vi "Read INI Cluster.vi"(8 "error in (no error)":errorcluster, 10 "INI Fomatted Cluster Type":variant, 11 "refnum":T1) -> (0 "error out":errorcluster, 1 "all found?":bool, 2 "INI Fomatted Cluster":variant, 3 "dup refnum":T1, 4 "any found?":bool)   [LabVIEW 2020]
doc: "Reads a cluster of section formatted clusters from configuration data identified by refnum, and returns them as a cluster of clusters of items. Section cluster names are used as section names and key-value pairs correspond to the named cluster elements and thier values within the section formatted clusters. Only the section clusters and items within the \"INI Formatted Cluster Type\" input cluster are read from the configuration data and returned in the output cluster of clusters of items. The \"found?\" output will be TRUE only if all elements (recursively) are found.\n\nFor example an Cluster containins subClusters MyCluster1 and MyCluster2, where MyCluster1 contains two elements MyNumeric and MyBoolean, and MyCluster2 contains two elements MyEnum and MyString. This would correspond to an INI write of the following data:\n\n[MyCluster1]\nMyNumeric=1.024\nMyBoolean=TRUE\n[MyCluster2]\nMyEnum=init\nMyString=\"Hello World\"\n\nNote: Special characters in section and key names will be escape-coded. These include the following: \\00-\\1F (non-printable chars); \"[\", \"]\", and \"=\" (INI syntax elements); \\FE (\"þ\") and \\FF (\"ÿ\") (legacy bracket encoding); Additionally, the escape character, \"\\\", will be escaped as \"\\\\\".\n\nNote: This VI checks whether every element of the cluster has a name so it can be identified."
uses:
  <vilib>/Utility/config.llb/Config Data RefNum.ctl
  <vilib>/Utility/config.llb/NI_LVConfig.lvlib
panel:
  # "Read INI Cluster.vi\n\nReads a cluster (variant) of INI section clusters from INI file.\n\nPlease visit http://www.OpenG.org to learn about the\nOpen Source LabVIEW software movement.\n\nNOTICE -- YOU MUST LEAVE THIS NOTICE IN PLACE.  PER THE TERMS OF THE LICENSE BELOW, YOU MAY SUBLICENSE THIS SOFTWARE \nIN ANY WAY THAT DOES NOT CONFLICT WITH THIS LICENSE.\n\n### BSD License (http://www.opensource.org/licenses/bsd-license.php) Begin ###\n \nCopyright (c) 2002-2006, Jim Kring <jim@jimkring.com>\n\nAll rights reserved.\n\nRedistribution and use in source and binary forms, with or without modification, are permitted provided that the following conditions are met:\n\n    * Redistributions of source code must retain the above copyright notice, this list of conditions and the following disclaimer.\n    * Redistributions in binary form must reproduce the above copyright notice, this list of conditions and the following disclaimer in the \n       documentation and/or other materials provided with the distribution.\n    * Neither the name of SciWare, James Kring, Inc., nor the names of its contributors may be used to endorse or promote products derived \n       from this software without specific prior written permission.\n\nTHIS SOFTWARE IS PROVIDED BY THE COPYRIGHT HOLDERS AND CONTRIBUTORS \"AS IS\" AND ANY EXPRESS OR IMPLIED WARRANTIES, \nINCLUDING, BUT NOT LIMITED TO, THE IMPLIED WARRANTIES OF MERCHANTABILITY AND FITNESS FOR A PARTICULAR PURPOSE ARE \nDISCLAIMED. IN NO EVENT SHALL THE COPYRIGHT OWNER OR CONTRIBUTORS BE LIABLE FOR ANY DIRECT, INDIRECT, INCIDENTAL,\n SPECIAL, EXEMPLARY, OR CONSEQUENTIAL DAMAGES (INCLUDING, BUT NOT LIMITED TO, PROCUREMENT OF SUBSTITUTE GOODS OR \nSERVICES; LOSS OF USE, DATA, OR PROFITS; OR BUSINESS INTERRUPTION) HOWEVER CAUSED AND ON ANY THEORY OF LIABILITY, \nWHETHER IN CONTRACT, STRICT LIABILITY, OR TORT (INCLUDING NEGLIGENCE OR OTHERWISE) ARISING IN ANY WAY OUT OF THE USE \nOF THIS SOFTWARE, EVEN IF ADVISED OF THE POSSIBILITY OF SUCH DAMAGE.\n\n### BSD License End ###"
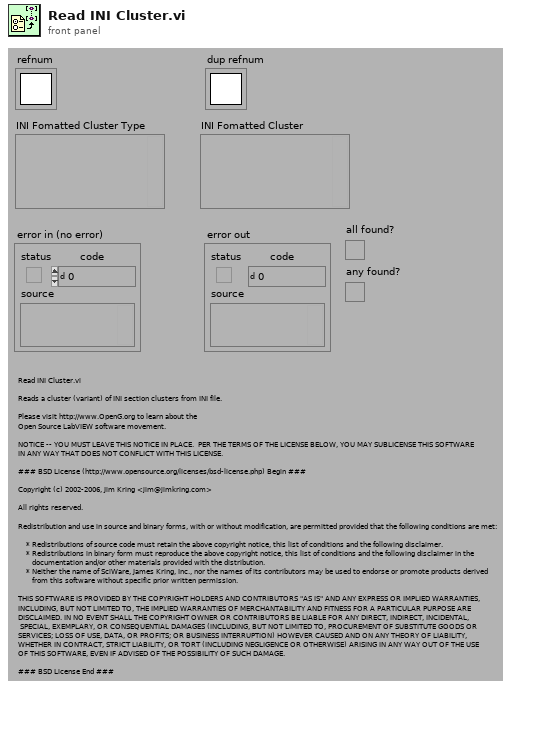
[diagram p1: front panel]
types:
  T1 = typedef "NI_LVConfig.lvlib/Config Data RefNum.ctl" = refnum<k1>
  T2 = typedef "Type Descriptor Enumeration.ctl" = enum8{"<Null>", "I8", "I16", "I32", "I64", "U8", "U16", "U32", "U64", "SGL", "DBL", "EXT", "CSG", "CDB", "CXT", "0x0F", "0x10", "0x11", "0x12", "0x13", "0x14", "Enum U8", "Enum U16", "Enum U32", "Enum U64", "SGL PQ", "DBL PQ", "EXT PQ", "CSG PQ", "CDB PQ", "CXT PQ", "0x1F", "0x20", "Boolean", "0x22", "0x23", "0x24", "0x25", "0x26", "0x27", "0x28", "0x29", "0x2A", "0x2B", "0x2C", "0x2D", "0x2E", "0x2F", "String", "0x31", "Path", "Pict", "0x34", "0x35", "0x36", "DAQ", "0x38", "0x39", "0x3A", "0x3B", "0x3C", "0x3D", "0x3E", "0x3F", "Array", "0x41", "0x42", "0x43", "0x44", "0x45", "0x46", "0x47", "0x48", "0x49", "0x4A", "0x4B", "0x4C", "0x4D", "0x4E", "0x4F", "Cluster", "0x51", "0x52", "Variant", "Waveform", "0x55", "0x56", "0x57", "0x58", "0x59", "0x5A", "0x5B", "0x5C", "0x5D", "0x5E", "0x5F", "0x60", "0x61", "0x62", "0x63", "0x64", "0x65", "0x66", "0x67", "0x68", "0x69", "0x6A", "0x6B", "0x6C", "0x6D", "0x6E", "0x6F", "Refnum"}
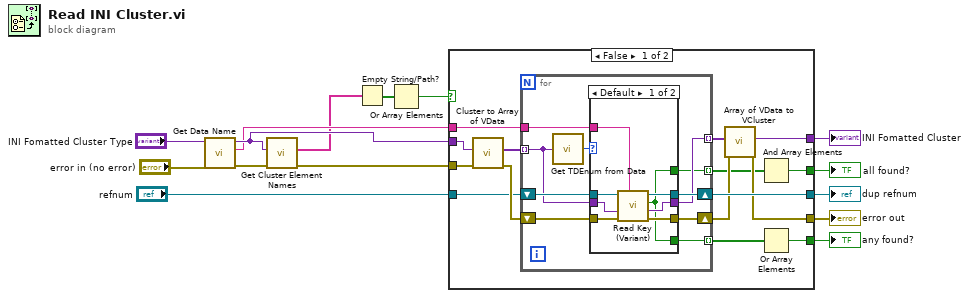
[diagram p0: block diagram]
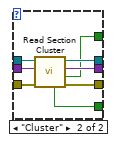
[diagram p2: hidden frame]
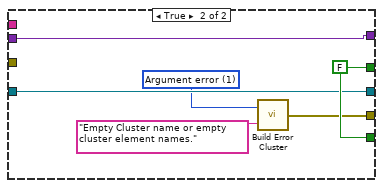
[diagram p3: hidden frame]
diagram:
  n1 = call "Get Data Name.vi"("error in (no error)"="error in (no error)", "Data"="INI Fomatted Cluster Type") -> ("error out"=w5:errorcluster, "Data Name"=w4:string, "Data dup"=w6:variant)  [unwired: 7 in]
  n2 = call "Get Cluster Element Names.vi"("error in (no error)"=w5, "Cluster"=w6) -> ("error out"=w2:errorcluster, "Element Names"=w1:string[])  [unwired: 8 in]
  n3 = Empty String/Path?(string/path=w1) -> (empty?=w7:bool[])
  n4 = Or Array Elements(Boolean array=w7) -> (logical OR=w3:bool)
  n5 = case shown="False" w3 {
    tunnel: [w29 w60] -> w15
    tunnel: "refnum" -> [w28 w60]
    tunnel: [w25 w62] -> w13
    tunnel: [w23 w57] -> w10
    tunnel: [w22 w61] -> w9
    tunnel: [w21 w61] -> w8
    tunnel: w6 -> [w18 w62]
    tunnel: w4 -> [w17 _]
    tunnel: w2 -> [w16 _]
    frame False {
      n6 = call "Cluster to Array of VData.vi"("error in (no error)"=w16, "Cluster"=w18) -> ("error out"=w30:errorcluster, "Array of VData"=w27:variant[])  [unwired: 8 in]
      n7 = for {
        tunnel: w27 -> [w35] mode=indexing
        shift-right: [w37] -> w29
        shift-left: w28 -> [w40]
        shift-right: [w38] -> w24
        shift-left: w30 -> [w39]
        tunnel: [w36] -> w26 mode=indexing
        tunnel: w17 -> [w33]
        tunnel: [w32] -> w19 mode=indexing
        tunnel: [w31] -> w20 mode=indexing
        n8 = call "Get TDEnum from Data.vi"("Data"=w35) -> ("Type Descriptor Enumeration"=w34:T2)  [unwired: 4 in]
        n9 = case shown="Default" w34 {
          tunnel: w40 -> [w46 w56]
          tunnel: w39 -> [w48 w55]
          tunnel: [w47 w54] -> w38
          tunnel: [w43 w53] -> w37
          tunnel: [w44 w52] -> w36
          tunnel: w35 -> [w42 w51]
          tunnel: w33 -> [w45 _]
          tunnel: [w41 w50] -> w32
          tunnel: [w41 w49] -> w31
          frame Default {
            n10 = call "Read Key (Variant).vi"("section"=w45, "error in (no error)"=w48, "type"=w42, "refnum"=w46) -> ("error out"=w47:errorcluster, "key-value"=w44:variant, "found?"=w41:bool, "refnum out"=w43:T1)  [unwired: 4 in]
          }
          frame "Cluster" {
            n11 = call "Read Section Cluster.vi"("error in (no error)"=w55, "Section Formatted Cluster Type"=w51, "refnum"=w56) -> ("error out"=w54:errorcluster, "all found?"=w50:bool, "Section Formatted Cluster"=w52:variant, "dup refnum"=w53:T1, "any found?"=w49:bool)  [unwired: 4 in]
          }
        }
      }
      n12 = call "Array of VData to VCluster.vi"("error in (no error)"=w24, "Array"=w26) -> ("error out"=w23:errorcluster, "VCluster"=w25:variant)  [unwired: 8 in]
      n13 = And Array Elements(Boolean array=w19) -> (logical AND=w22:bool)
      n14 = Or Array Elements(Boolean array=w20) -> (logical OR=w21:bool)
    }
    frame True {
      w59 = 1 items=["No error", "Argument error", "Memory is full", "Out of zone", "End of file", "File already open", "Generic file I/O error", "File not found", "File permission error", "Disk is full", "Duplicate path", "Too many files open", "System feature not enabled", "Resource file not found", "Cannot add resource", "Resource not found", "Image not found", "Image memory error", "Pen does not exist", "Config type invalid", "Config token not found", "Config parse error", "Config memory error", "Bad external code format", "Bad external code offset", "External code not present", "Null window", "Destroy window error", "Null menu", "Print aborted", "Bad print record", "Print driver error", "Windows error during printing", "Memory error during printing", "Print dialog error", "Generic print error", "Invalid device refnum", "Device not found", "Device parameter error", "Device unit error", "Cannot open device", "Device call aborted", "Generic error", "Cancelled by user", "Object ID too low", "Object ID too high", "Object not in heap", "Unknown heap", "Unknown object (invalid DefProc)", "Unknown object (DefProc not in table)", "Message out of range", "Invalid (null) method", "Unknown message", "Manager call not supported", "Bad address", "Network operation in progress", "Network operation timed out", "Connection is busy", "Network attribute not supported", "Network error", "Address in use", "System out of memory", "Connection aborted", "Connection refused", "Not connected", "Already connected", "Connection closed", "Initialization error (interapplication manager)", "Bad occurrence", "Wait on unbound occurrence handler", "Occurrence queue overflow", "Datalog type conflict", "Unused", "Unrecognized type (interapplication manager)", "Memory corrupt", "Failed to make temporary DLL", "Old CIN version", "Drag socket not found", "Failed to load drop-object", "Failed to register OLE object", "Failed to release OLE object", "Format specifier type mismatch", "Unknown format specifier", "Too few format specifiers", "Too many format specifiers", "Scan failed", "Newer CIN version", "Error converting to variant", "Runtime menu error", "Password tampered", "Variant attribute not found", "Incompatible variant data type", "Event data is not available", "Event Store is not present", "Occurrence is not found", "Event Queue is not created", "Event info is not available", "Refnum passed is NULL", "Error retrieving Class GUID", "Error retrieving CoClass GUID", "Error retrieving TypeLib GUID.", "Bad built application magic bytes.", "Specific driver is different from the specific driver associated with the Logical Name.", "There is no session opened to the class driver.", "Max Error", "MAX - Error with config objects", "MAX - Error loading configuration", "MAX - Group not supported"]
      w61 = FALSE
      n15 = call "Build Error Cluster.vi"("String to Prepend to source (\"\")"="Empty Cluster name or empty cluster element names." ("String to Prepend to source (\"\")"), "code"=w59) -> ("error out"=w57:errorcluster)
    }
  }
  "error out" <- w10
  "dup refnum" <- w15
  "INI Fomatted Cluster" <- w13
  "all found?" <- w9
  "any found?" <- w8
